vi "Get Column Headers.vi"(8 "error in (no error)":errorcluster, 11 "DataGrid Config in":refnum<class "DataGrid Config.lvclass">) -> (0 "error out":errorcluster, 2 "Column Headers[]":string[](array[string]), 3 "DataGrid Config out":refnum<class "DataGrid Config.lvclass">)   [LabVIEW 2018, in "DataGrid Config.lvclass"]
uses:
  DataGrid Config.lvclass
  DataGrid Config.lvclass/DataGrid Config.ctl
  Data Type Classes/Generic/Generic Data Type.lvclass/Generic Data Type.ctl
  Data Type Classes/Generic/Read Column Header.vi
  Data Type Classes/Generic/Generic Data Type.lvclass
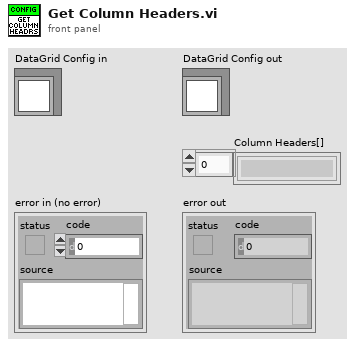
[diagram p1: front panel]
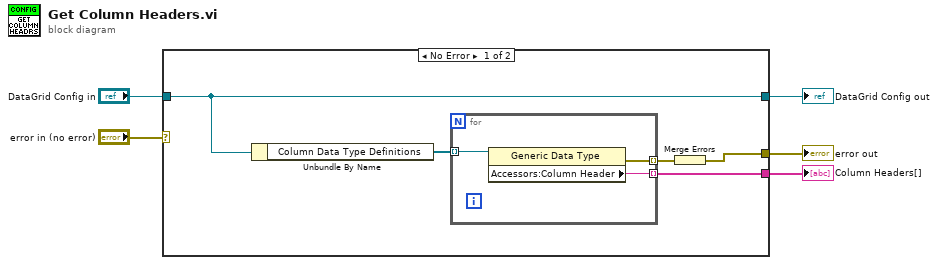
[diagram p0: block diagram]
diagram:
  n1 = case shown="No Error" "error in (no error)" {
    selector: "error in (no error)" -> [_ w15]
    tunnel: [w6 w15] -> w4
    tunnel: [w10 w14] -> w2
    tunnel: "DataGrid Config in" -> [w10 w14]
    tunnel: [w8 _] -> w1
    frame No Error {
      n2 = Unbundle By Name(w10) -> ("Column Data Type Definitions"=w9:refnum<class "Generic Data Type.lvclass">[])
      n3 = for {
        tunnel: w9 -> [w13] mode=indexing
        tunnel: [w12] -> w8 mode=indexing
        tunnel: [w11] -> w7 mode=indexing
        n4 = property class="Generic Data Type"(reference=w13) -> (error out=w11:errorcluster, "Accessors:Column Header"=w12:string)  [unwired: 1 in, 1 out]
      }
      n5 = Merge Errors(w7) -> (w6:errorcluster)
    }
    frame Error {
    }
  }
  "error out" <- w4
  "DataGrid Config out" <- w2
  "Column Headers[]" <- w1
